vi "Compare Variants.vi"(6 "Delta":variant, 8 "error in (no error)":errorcluster, 9 "Actual":variant, 10 "Expected":variant) -> (0 "error out":errorcluster, 2 "Equal?":bool)   [LabVIEW 2020]
uses:
  LUnit Inheriting Test Case.lvclass/LUnit Inheriting Test Case.ctl
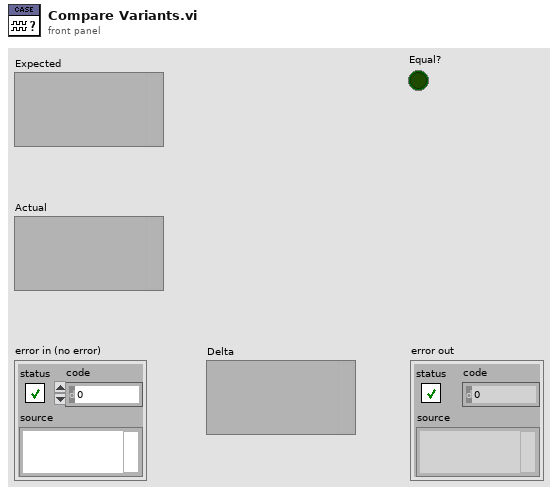
[diagram p1: front panel]
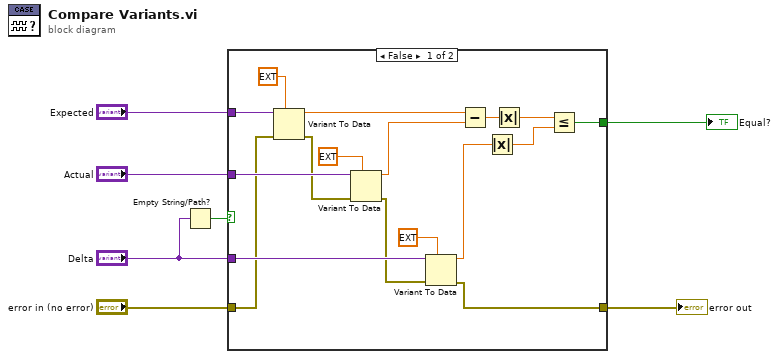
[diagram p0: block diagram]
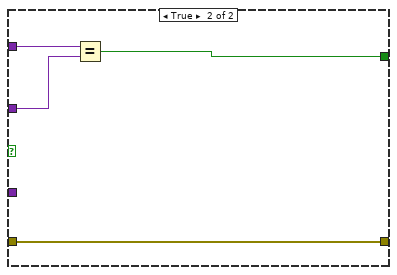
[diagram p2: hidden frame]
diagram:
  n1 = Empty String/Path?(string/path="Delta") -> (empty?=w1:bool)
  n2 = case shown="False" w1 {
    tunnel: "Delta" -> [w24 _]
    tunnel: "Expected" -> [w22 w28]
    tunnel: "Actual" -> [w23 w27]
    tunnel: [w14 w25] -> w4
    tunnel: [w9 w26] -> w5
    tunnel: "error in (no error)" -> [w8 w25]
    frame False {
      n3 = Variant To Data(error in=w8, type=ext 0.0, Variant=w22) -> (data=w13:ext, error out=w16:errorcluster)
      n4 = Variant To Data(error in=w16, type=ext 0.0, Variant=w23) -> (data=w12:ext, error out=w15:errorcluster)
      n5 = Variant To Data(error in=w15, type=ext 0.0, Variant=w24) -> (data=w11:ext, error out=w14:errorcluster)
      n6 = Subtract(x=w13, y=w12) -> (x-y=w19:ext)
      n7 = Absolute Value(x=w11) -> (abs(x)=w10:ext)
      n8 = Absolute Value(x=w19) -> (abs(x)=w18:ext)
      n9 = Less Or Equal?(x=w18, y=w10) -> (x <= y?=w9:bool)
    }
    frame True {
      n10 = Equal?(x=w28, y=w27) -> (x = y?=w26:bool)
    }
  }
  "Equal?" <- w5
  "error out" <- w4
